vi "Add Comment.vi"(8 "Error In":errorcluster, 10 "Comment":string, 11 "Message In":string) -> (0 "Error Out":errorcluster, 3 "Message Out":string)   [LabVIEW 2014, in "i3-sse-server.lvlib"]
uses:
  i3-sse-server.lvlib
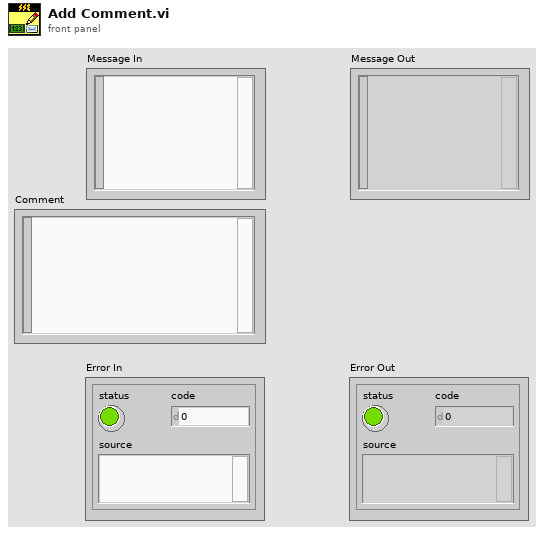
[diagram p1: front panel]
types:
  T1 = enum16{"Native", "Native Command Line", "UNIX", "Macintosh", "DOS"}
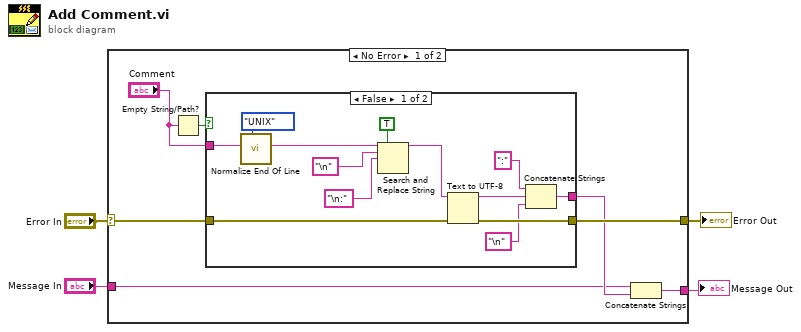
[diagram p0: block diagram]
diagram:
  n1 = case shown="No Error" "Error In" {
    selector: "Error In" -> [w9 w28]
    tunnel: [w8 w28] -> w2
    tunnel: [w7 w27] -> w3
    tunnel: "Message In" -> [w5 w27]
    frame No Error {
      n2 = Empty String/Path?(string/path="Comment") -> (empty?=w11:bool)
      n3 = case shown="False" w11 {
        tunnel: "Comment" -> [w24 w25]
        tunnel: w9 -> [w19 w26]
        tunnel: [w18 w26] -> w8
        tunnel: [w16 w25] -> w6
        frame False {
          n4 = call <vilib>:"Normalize End Of Line.vi"("end of line (Native)"=T1."UNIX", "string in"=w24) -> ("string out"=w12:string)  [unwired: 6 in]
          n5 = Search and Replace String(replace all?=TRUE ("replace all? (F)"), input string=w12, search string="\n", replace string="\n:" ("search string")) -> (result string=w17:string)  [unwired: 4 in, 3 out]
          n6 = Text to UTF-8(8:w19, 11:w17) -> (0:w18:errorcluster, 3:w14:string)  [unwired: 1 in]
          n7 = Concatenate Strings(":" ("string"), w14, "\n" ("string")) -> (w16:string)
        }
        frame True {
        }
      }
      n8 = Concatenate Strings(w5, w6) -> (w7:string)
    }
    frame Error {
    }
  }
  "Error Out" <- w2
  "Message Out" <- w3
